vi "Dashboard Main.vi"() -> ()   [LabVIEW 2013]
uses:
  <vilib>/event_ctls.llb/eventvkey.ctl
  <vilib>/Rock Robotics/WPI/Dashboard/WPI_DashboardLogging Global.vi
  <vilib>/Utility/config.llb/Write Key (String).vi
  <vilib>/Utility/config.llb/Write Key (I32).vi
  <vilib>/Utility/config.llb/NI_LVConfig.lvlib
panel:
  out "Image Message":string="Timeout in Camera Communications"
  in  "Rec Mode":enum32{"Stop", "Record", "Playback"}(radio)
  in  "Dashboard Tab":T1(tab)
  in  "Camera Settings":T2={"Frame Rate"=30, "Compression"=30, "Size"=1} {"Frame Rate" scale=1.0..30.0; "Size" items=["640x480", "320x240", "160x120"]}
  out "MotorSliders R":cluster{"MotorSlide1":dbl, "MotorSlide2":dbl} {"MotorSlide2" scale=-1.0..1.0 scale format="%#_2e"; "MotorSlide1" scale=-1.0..1.0 scale format="%#_2e"}
  out "MotorChart R":cluster{"Numeric":dbl, "Numeric":dbl}(graph)
  out "MotorSliders L":T3 {"MotorSlide4 2" scale=0.0..14.0 scale format="%#_2e"; "MotorSlide2" scale=-1.0..1.0 scale format="%#_2e"; "MotorSlide1" scale=-1.0..1.0 scale format="%#_2e"}
  out "MotorChart L":T4(graph)
  out "JS1 Z":dbl(slide) scale=-1.0..1.0 scale format="%#_2e"
  out "Joystick 1":cluster{"X":dbl, "Y":dbl}[](graph)
  out "JS Buttons 1":T5
  out "JS2 Z":dbl(slide) scale=-1.0..1.0 scale format="%#_2e"
  out "Joystick 2":cluster{"X":dbl, "Y":dbl}[](graph)
  out "JS Buttons 2":T5
  out "Mode":T6(ring)=enum."Auto Disabled"
  out "Camera IP":string
  in  "DB Camera Config":bool
  out "fps":dbl format="%#.1g"
  out "Mbps":dbl format="%#.1g"
  out "Mbps 2":bool
  out "LED 1":bool
  in  "Slider 1":dbl(slide) scale=0.0..100.0
  in  "Checkbox 2":bool
  in  "Checkbox 1":bool
  in  "Test Slider":dbl(slide) scale=0.0..100.0 scale format="%#_3g"
  in  "On/Off":bool caption="Solenoid"
  in  "Test Name":u16(ring) items=["Select the test to run...", "Example Test", "-------------------------------", "List of tests is built in robot code.", "Replace with your own automated tests."]
  in  "Test Tree":string(tree)
  in  "Motor":cluster{"Value":dbl, "Enable":bool} {"Value" scale=-1.0..1.0 scale format="%#_3g"}
  out "Progress":T7 {"Test Progress" scale=0.0..100.0}
  in  "Rev/Fwd":cluster{"Forward":bool, "Reverse":bool}
  in  "Test Ring":u16(ring) items=["Auto", "Fixed indoor", "Fixed outdoor 1", "Fixed outdoor 2", "Fixed fluorescent 1", "Fixed fluorescent 2", "Hold current"]
  in  "Listbox":i32(listbox)
  out "Tree":string(tree)
  out "Camera Image":T8(plugin-control)
  in  "Enable":bool
  # "Left"
  # "Front"
  # "Right"
  # "Battery"
  # "Customize by placing controls and indicators here and name to\nmatch Dashboard Variables on robot."
  # "This tab is a great place for autonomous settings and validation.\nCustomize by placing controls and indicators here and name to\nmatch Dashboard Variables on robot."
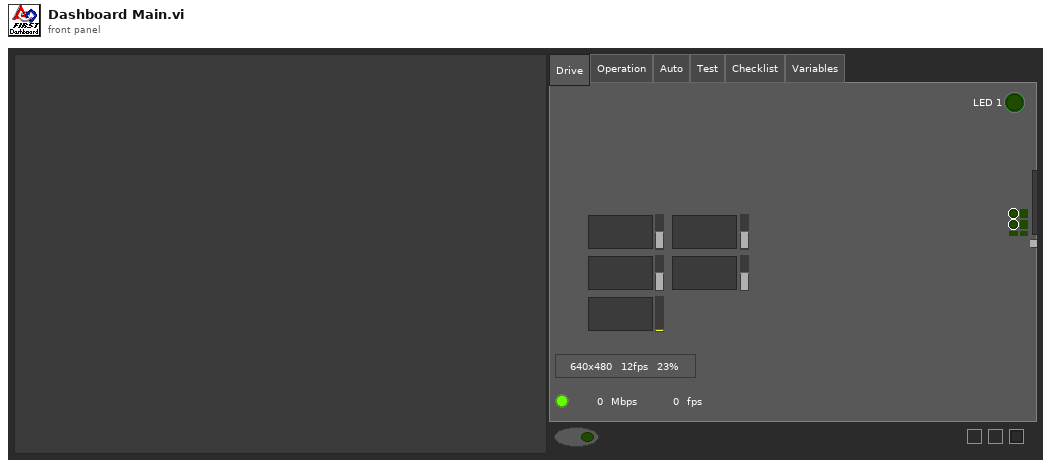
[diagram p1: front panel]
types:
  T1 = enum32{"Drive", "Operation", "Auto", "Test", "Checklist", "Variables"}
  T2 = cluster{"Frame Rate":i32, "Compression":i32, "Size":u16}
  T3 = cluster{"MotorSlide1":dbl, "MotorSlide2":dbl, "MotorSlide4 2":dbl}
  T4 = cluster{"Numeric":dbl, "Numeric":dbl, "Battery":sgl}
  T5 = cluster{bool, bool, bool, bool, bool, bool, bool, bool, bool, bool, bool, bool}
  T6 = enum8{"Tele-Op Disabled", "Tele-Op Enabled", "Auto Disabled", "Auto Enabled", "Test Disabled", "Test Enabled", ""}
  T7 = cluster{"Test Progress":u8, "Test Progress Text":string}
  T8 = typedef "IMAQ Image.ctl" = refnum<image>
  T9 = typedef "Image Type" = u32
  T10 = cluster{"Digital Inputs":bool[], "Digital Outputs":bool[]}
  T11 = cluster{"Competition mode":bool, "Robot Link":bool, "Autonomous":bool, "Enabled":bool, "E-Stop":bool, "Simulated":bool, "TestMode":bool, "Docked Window":bool}
  T12 = enum16{"0", "1", "2", "3", "4", "5", "6", "7", "8", "9", "A", "B", "C", "D", "E", "F", "G", "H", "I", "J", "K", "L", "M", "N", "O", "P", "Q", "R", "S", "T", "U", "V", "W", "X", "Y", "Z", "F1", "F2", "F3", "F4", "F5", "F6", "F7", "F8", "F9", "F10", "F11", "F12", "F13", "F14", "F15", "ADD", "BACK", "BACKSLASH", "CAPITAL", "COMMA", "DECIMAL", "DELETE", "DIVIDE", "DOWN", "END", "EQUALS", "ESCAPE", "GRAVE (`)", "HOME", "INSERT", "LBRACKET", "LCONTROL", "LEFT", "L ALT", "LSHIFT", "LWIN", "MINUS", "MULTIPLY", "NEXT", "NUMLOCK", "NUMPAD_0", "NUMPAD_1", "NUMPAD_2", "NUMPAD_3", "NUMPAD_4", "NUMPAD_5", "NUMPAD_6", "NUMPAD_7", "NUMPAD_8", "NUMPAD_9", "PAUSE", "PERIOD", "PRIOR (PG UP)", "RBRACKET", "RCONTROL", "RETURN", "RIGHT", "R ALT", "RSHIFT", "RWIN", "SCROLL", "SEMICOLON", "SLASH", "SPACE", "SUBTRACT", "TAB", "UP", "ENTER (num pad)", "' (quote)"}
  T13 = cluster{"Boolean Array[0]":bool, "Boolean Array[1]":bool, "Boolean Array[2]":bool, "Boolean Array[3]":bool, "Boolean Array[4]":bool, "Boolean Array[5]":bool, "Boolean Array[6]":bool, "Boolean Array[7]":bool, "Boolean Array[8]":bool, "Boolean Array[9]":bool, "Boolean Array[10]":bool, "Boolean Array[11]":bool}
  T14 = typedef "NI_LVConfig.lvlib/Config Data RefNum.ctl" = refnum<k1>
  T15 = typedef "eventvkey.ctl" = enum16{"ASCII", "Enter", "Return", "Shift", "Ctrl", "Alt", "Cmd", "Opt", "Caps", "NumLock", "Clear", "Break", "Up", "Down", "Left", "Right", "Insert", "Delete", "Home", "End", "PageUp", "PageDown", "Escape", "Help", "Pause", "ScrollLock", "F1", "F2", "F3", "F4", "F5", "F6", "F7", "F8", "F9", "F10", "F11", "F12", "F13", "F14", "F15", "F16", "F17", "F18", "F19", "F20", "F21", "F22", "F23", "F24", "Play", "VolumeUp", "VolumeDown", "Mute", "Two Byte Char"}
  T16 = cluster{"Image Size":bool, "Image Type":bool, "Pixel Value":bool, "ROI Information":bool, "Zoom Factor":bool}
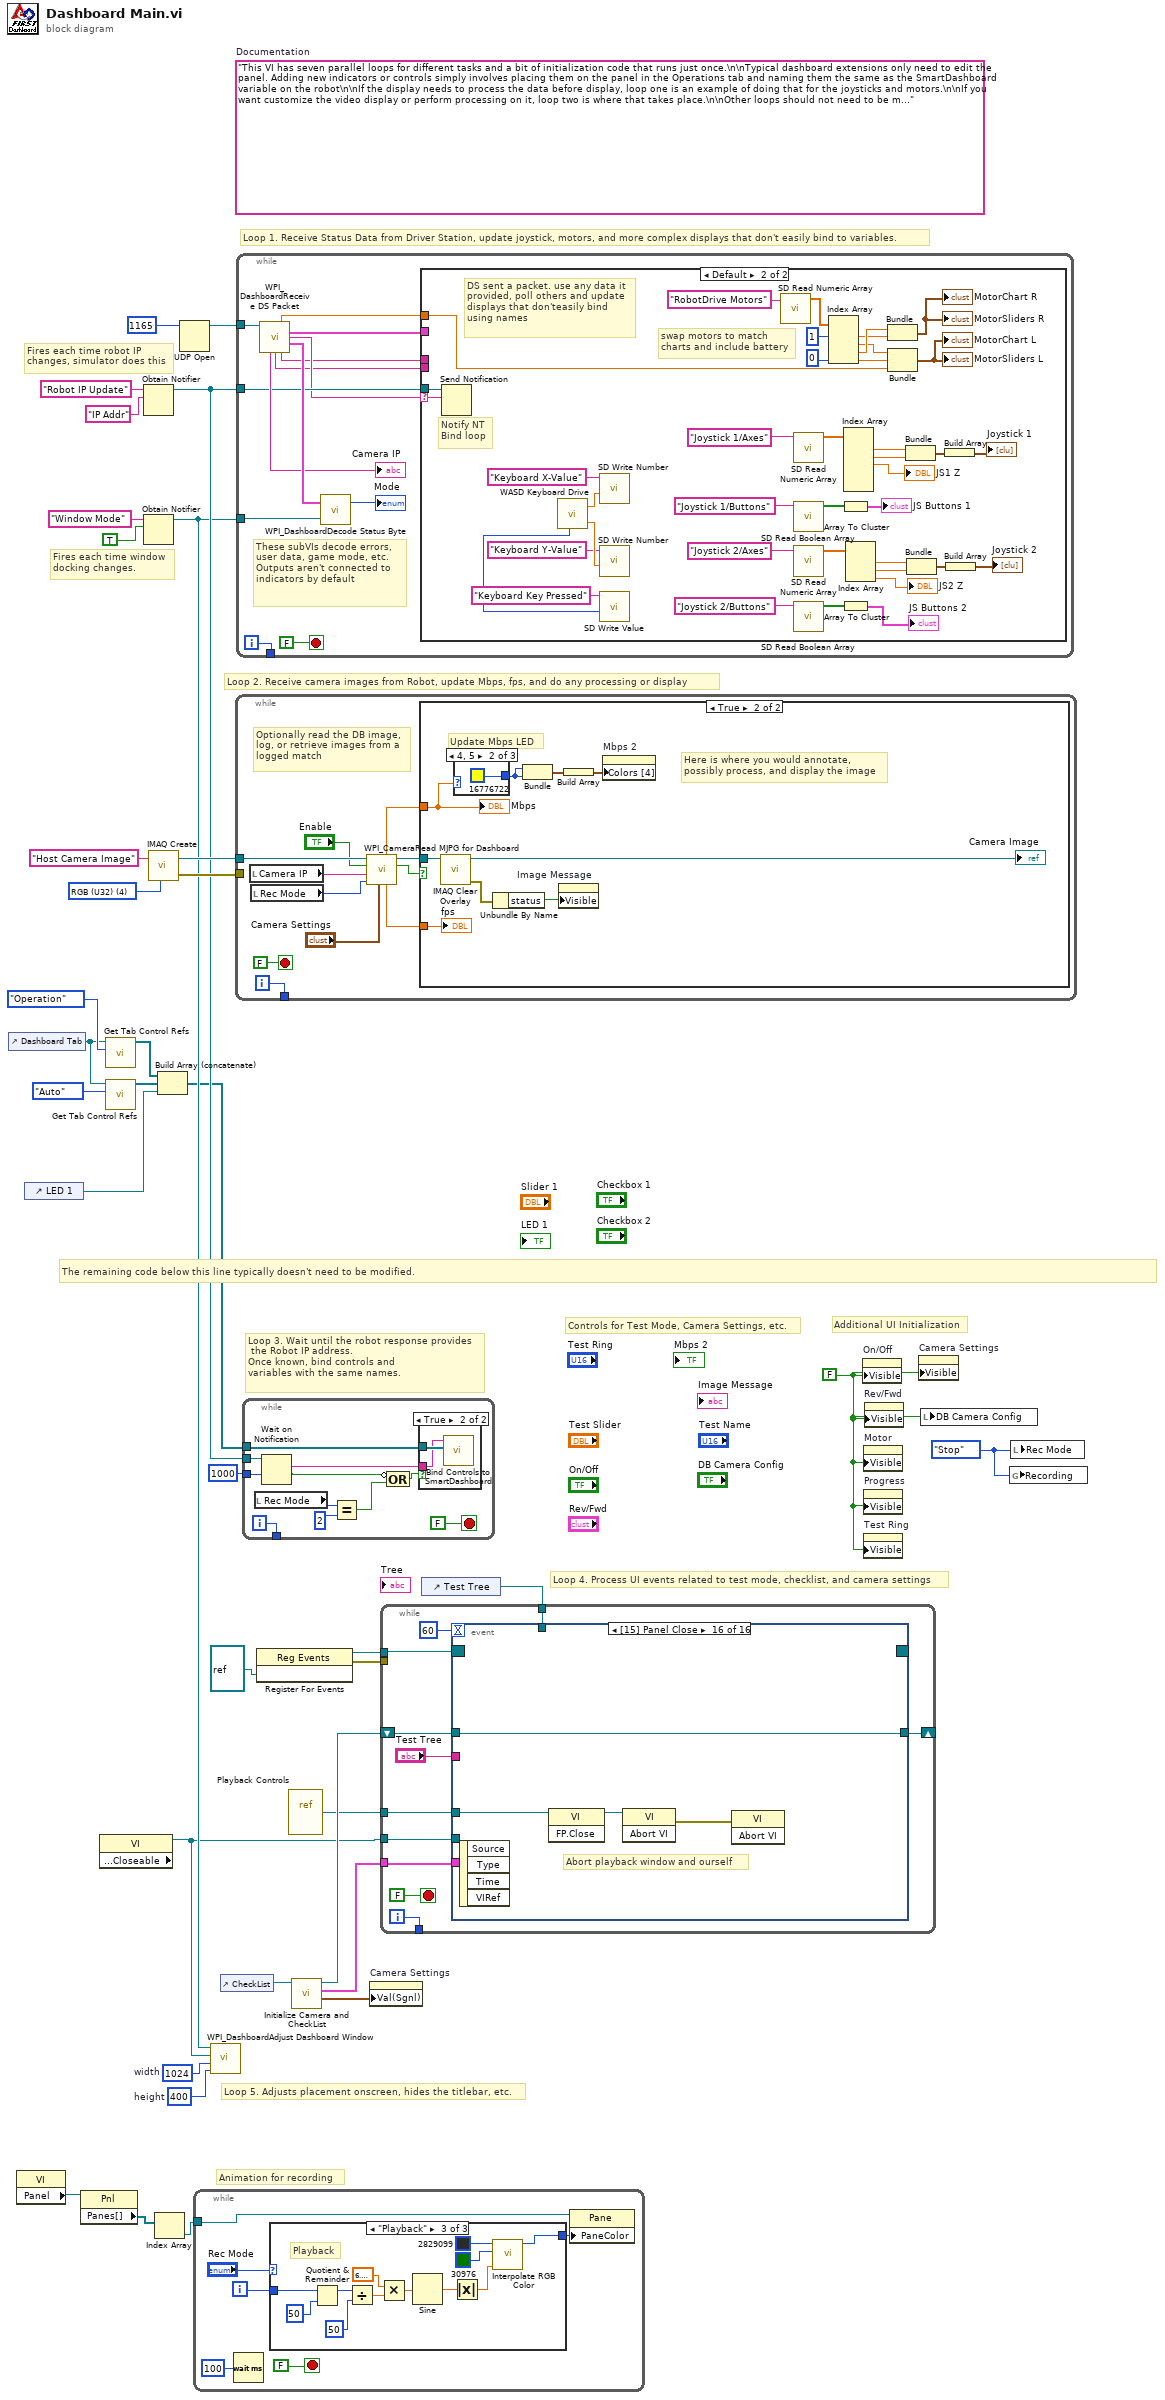
[diagram p0: block diagram]
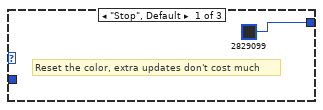
[diagram p2: hidden frame]
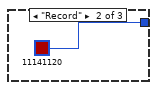
[diagram p3: hidden frame]
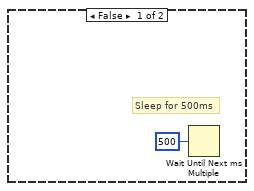
[diagram p5: hidden frame]
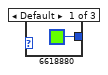
[diagram p6: hidden frame]
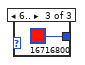
[diagram p7: hidden frame]
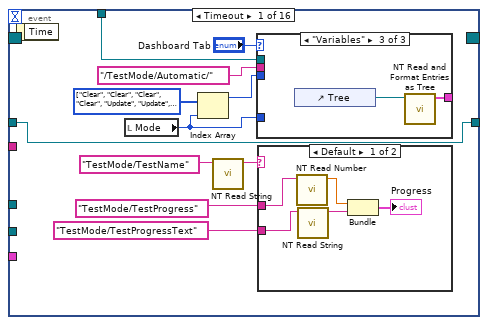
[diagram p8: hidden frame]
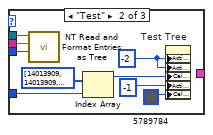
[diagram p10: hidden frame]
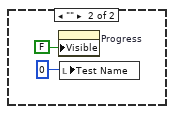
[diagram p11: hidden frame]
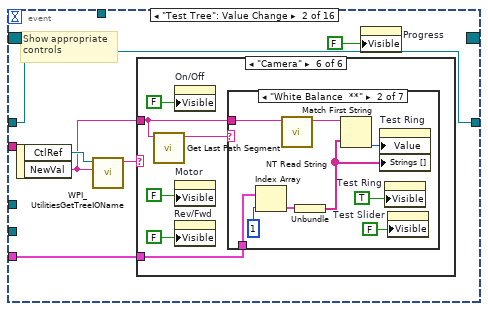
[diagram p12: hidden frame]
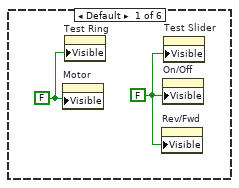
[diagram p13: hidden frame]
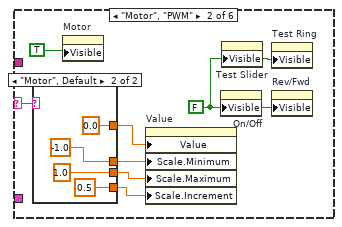
[diagram p14: hidden frame]
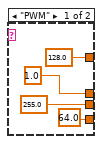
[diagram p15: hidden frame]
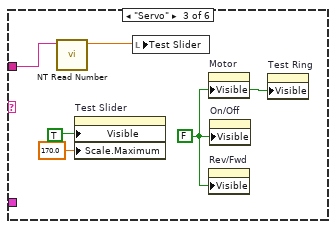
[diagram p16: hidden frame]
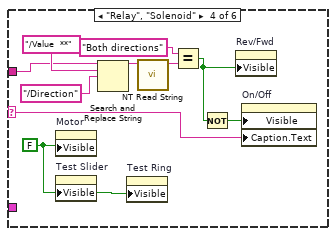
[diagram p17: hidden frame]
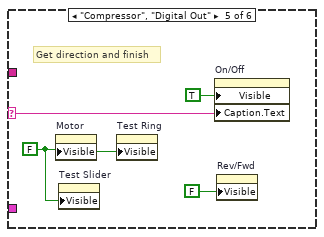
[diagram p18: hidden frame]
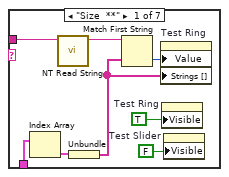
[diagram p19: hidden frame]
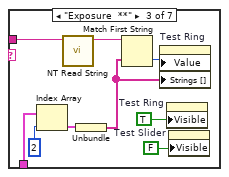
[diagram p20: hidden frame]
diagram:
  w8 = enum32{"Stop", "Record", "Playback"}."Stop" ("Rec Mode")
  w11 = 400  # height
  w12 = 1024  # width
  w25 = FALSE ("Visible")
  (unwired) "This VI has seven parallel loops for different tasks and a bit of initialization code that runs just once.\n\nTypical dashboard extensions only need to edit the panel. Adding new indicators or controls simply involves placing them on the panel in the Operations tab and naming them the same as the SmartDashboard variable on the robot\n\nIf the display needs to process the data before display, loop one is an example of doing that for the joysticks and motors.\n\nIf you want customize the video display or perform processing on it, loop two is where that takes place.\n\nOther loops should not need to be modified. They are pretty standard, and document the task they perform."  # Documentation
  w35 = T9 4 items=["Grayscale (U8)", "Grayscale (I16)", "Grayscale (SGL)", "Complex (CSG)", "RGB (U32)", "HSL (U32)", "RGB (U64)"] ("Image Type")
  # "Controls for Test Mode, Camera Settings, etc."
  # "Additional UI Initialization"
  # "Animation for recording"
  # "Fires each time robot IP\nchanges, simulator does this"
  # "Fires each time window\ndocking changes."
  # "The remaining code below this line typically doesn't need to be modified."
  # "Loop 4. Process UI events related to test mode, checklist, and camera settings"
  # "Loop 3. Wait until the robot response provides\n the Robot IP address.\nOnce known, bind controls and\nvariables with the same names."
  # "Loop 5. Adjusts placement onscreen, hides the titlebar, etc."
  # "Loop 1. Receive Status Data from Driver Station, update joystick, motors, and more complex displays that don't easily bind to variables."
  # "Loop 2. Receive camera images from Robot, update Mbps, fps, and do any processing or display"
  n1 = control-ref of="Dashboard Tab"() -> (w6:refnum<vi>)
  n2 = property class="VI"() -> ("Panel"=w19:refnum<vi>)  [unwired: 2 in, 2 out]
  n3 = control-ref of="LED 1"() -> (w1:refnum<vi>)
  n4 = property class="Pnl"(reference=w19) -> ("Panes[]"=w20:refnum<vi>[])  [unwired: 1 in, 2 out]
  n5 = property class="VI" props=["Front Panel.Closeable"]() -> (reference out=w7:refnum<vi>)  [unwired: 2 in, 2 out]
  n6 = call <vilib>:"Get Tab Control Refs.vi"("Page Index"=T1."Operation" ("Dashboard Tab"), "TabControl in"=w6) -> ("ControlsOnPage"=w4:refnum<vi>[])  [unwired: 9 in]
  n7 = call <vilib>:"Get Tab Control Refs.vi"("Page Index"=T1."Auto" ("Dashboard Tab"), "TabControl in"=w6) -> ("ControlsOnPage"=w5:refnum<vi>[])  [unwired: 9 in]
  n8 = Obtain Notifier(name (unnamed)="Robot IP Update", notification data type="IP Addr" ("name (unnamed)")) -> (notifier out=w29:refnum<notifier>)  [unwired: 2 in, 2 out]
  n9 = Obtain Notifier(name (unnamed)="Window Mode", notification data type=TRUE) -> (notifier out=w10:refnum<notifier>)  [unwired: 2 in, 2 out]
  n10 = call "IMAQ Create"("Image Name"="Host Camera Image", "Image Type"=w35) -> ("New Image"=w33:T8, "error out"=w32:errorcluster)  [unwired: 2 in, 1 out]
  n11 = Index Array(array=w20) -> (element=w18:refnum<vi>)  [unwired: 1 in]
  n12 = Build Array (concatenate)(w4, w5, w1) -> (w3:refnum<vi>[])
  n13 = UDP Open(11:u16 1165 ("port")) -> (port=w36:refnum<k16>)  [unwired: 2 in, 4 out]
  n14 = while {
    tunnel: w18 -> [w39]
    i -> [w42]
    stop <- FALSE stop-if-true
    n15 = Wait (ms)(milliseconds to wait=u32 100) -> ()  [unwired: 1 out]
    n16 = case shown="\"Playback\"" "Rec Mode" {
      tunnel: w42 -> [_ _ w57]
      tunnel: [u32 2829099 ("Base Color") u32 11141120 ("Target Color") w46] -> w38
      frame "Stop", Default {
        # "Reset the color, extra updates don't cost much"
      }
      frame "Record" {
      }
      frame "Playback" {
        # "Playback"
        n17 = Quotient & Remainder(x=w57, y=u32 50 ("milliseconds to wait")) -> (x-y*floor(x/y)=w53:u32)  [unwired: 1 out]
        n18 = Divide(x=w53, y=u32 50 ("milliseconds to wait")) -> (x/y=w50:dbl)
        n19 = Multiply(x=6.283185307179586, y=w50) -> (x*y=w55:dbl)
        n20 = Sine(x=w55) -> (sin(x)=w54:dbl)
        n21 = Absolute Value(x=w54) -> (abs(x)=w47:dbl)
        n22 = call "Interpolate RGB Color.vi"("Proportion"=w47, "Target Color"=u32 30976, "Base Color"=u32 2829099) -> ("Result Color"=w46:u32)  [unwired: 8 in]
      }
    }
    n23 = property class="Pane"(reference=w39, "PaneColor"=w38) -> ()  [unwired: 1 in, 2 out]
  }
  n24 = call <vilib>:"WPI_DashboardAdjust Dashboard Window.vi"("height"=w11, "width"=w12, "reference in"=w7, "Notifier in"=w10) -> ()  [unwired: 8 in]
  n25 = control-ref of="CheckList"() -> (w9:refnum<vi>)
  n26 = while {
    tunnel: w33 -> [w66]
    tunnel: w32 -> [_]
    tunnel: [w67] -> _
    i -> [w67]
    stop <- FALSE stop-if-true
    # "Optionally read the DB image,\nlog, or retrieve images from a\nlogged match"
    n27 = local read "Camera IP"() -> (w59:string)
    n28 = local read "Rec Mode"() -> (w58:enum32{"Stop", "Record", "Playback"})
    n29 = call <vilib>:"WPI_CameraRead MJPG for Dashboard.vi"("Camera Settings"="Camera Settings", "Rec Mode"=w58, "Camera IP"=w59, "Enable"="Enable", "Refnum in"=w66) -> ("Active"=w63:bool, "Refnum out"=w65:T8, "FPS"=w62:dbl, "Bandwidth (Mbps)"=w61:dbl)  [unwired: 3 in]
    n30 = case shown="True" w63 {
      tunnel: w65 -> [_ w73]
      tunnel: w61 -> [_ w72]
      tunnel: w62 -> [_ w70]
      frame False {
        # "Sleep for 500ms"
        n31 = Wait Until Next ms Multiple(millisecond multiple=u32 500) -> ()  [unwired: 1 out]
      }
      frame True {
        # "Here is where you would annotate,\npossibly process, and display the image"
        # "Update Mbps LED"
        n32 = call "IMAQ Clear Overlay"("Image"=w73) -> ("error out"=w77:errorcluster, "Image Out"=→"Camera Image":T8)  [unwired: 2 in, 7 out]
        n33 = case shown="4, 5" w72 {
          tunnel: [u32 6618880 ("Color Box") u32 16776722 ("Color Box") u32 16716800 ("Color Box")] -> w74
          frame Default {
          }
          frame 4, 5 {
          }
          frame 6.. {
          }
        }
        n34 = Unbundle By Name(w77) -> ("status"=w78:bool)
        n35 = Bundle("Color Box"=w74, "Color Box"=w74) -> (w76:cluster{"Color Box":u32, "Color Box":u32})  [unwired: 1 out]
        n36 = property on="Image Message" class="Str"("Visible"=w78) -> ()  [unwired: 2 in, 2 out]
        n37 = Build Array(w76) -> (w75:cluster{"Color Box":u32, "Color Box":u32}[])
        n38 = property on="Mbps 2" class="Bool (strict)"("Colors [4]"=w75) -> ()  [unwired: 2 in, 2 out]
        "Mbps" <- w72
        "fps" <- w70
      }
    }
  }
  n39 = while {
    tunnel: w36 -> [w92]
    tunnel: w29 -> [w87]
    tunnel: w10 -> [w91]
    tunnel: [w88] -> _
    i -> [w88]
    stop <- FALSE stop-if-true
    # "These subVIs decode errors, user data, game mode, etc.\nOutputs aren't connected to indicators by default"
    n40 = call <vilib>:"WPI_DashboardReceive DS Packet.vi"("Recv Socket"=w92) -> ("Battery"=w82:sgl, "Driver Station"=w83:T10, "Robot IP Address"=w86:string, "Status"=w93:T11, "Camera IP Address"=→"Camera IP":string, "Low Priority User Data"=w85:string, "High Priority User Data"=w84:string)  [unwired: 1 in, 7 out]
    n41 = call <vilib>:"WPI_DashboardDecode Status Byte.vi"("Window Mode Notifier"=w91, "Status"=w93) -> ("Mode"=→"Mode":T6)  [unwired: 1 out]
    n42 = case shown="Default" w86 {
      selector: w86 -> [_ w111]
      tunnel: w87 -> [_ w112]
      tunnel: w85 -> [_ _]
      tunnel: w84 -> [_ _]
      tunnel: w83 -> [_ _]
      tunnel: w82 -> [_ w110]
      frame "0.0.0.0" {
        # "DS not sending packets, or no robot exists yet.\nDon't poll the variables"
      }
      frame Default {
        # "Notify NT\nBind loop"
        # "DS sent a packet. use any data it\nprovided, poll others and update\ndisplays that don'teasily bind\nusing names"
        # "swap motors to match\ncharts and include battery"
        n43 = Send Notification(notification=w111, notifier=w112) -> ()  [unwired: 1 in, 2 out]
        n44 = call "WASD Keyboard Drive.vi"() -> ("Y-Axis"=w98:dbl, "X-Axis"=w100:dbl, "key"=w96:T12)  [unwired: 5 in]
        n45 = call <vilib>:"SD Write Number.vi"("Numeric"=w100, "Name"="Keyboard X-Value") -> ()  [unwired: 8 in, 2 out]
        n46 = call <vilib>:"SD Write Number.vi"("Numeric"=w98, "Name"="Keyboard Y-Value") -> ()  [unwired: 8 in, 2 out]
        n47 = call-poly <vilib>:"SD Write Value.vi"("Numeric"=w96, "Name"="Keyboard Key Pressed") -> ()  [unwired: 8 in, 2 out]
        n48 = call <vilib>:"SD Read Numeric Array.vi"("Name"="RobotDrive Motors") -> ("Numeric Array"=w109:dbl[])  [unwired: 8 in, 2 out]
        n49 = call <vilib>:"SD Read Numeric Array.vi"("Name"="Joystick 1/Axes") -> ("Numeric Array"=w128:dbl[])  [unwired: 8 in, 2 out]
        n50 = call <vilib>:"SD Read Boolean Array.vi"("Name"="Joystick 1/Buttons") -> ("Boolean Array"=w130:bool[])  [unwired: 8 in, 2 out]
        n51 = call <vilib>:"SD Read Numeric Array.vi"("Name"="Joystick 2/Axes") -> ("Numeric Array"=w122:dbl[])  [unwired: 8 in, 2 out]
        n52 = call <vilib>:"SD Read Boolean Array.vi"("Name"="Joystick 2/Buttons") -> ("Boolean Array"=w121:bool[])  [unwired: 8 in, 2 out]
        n53 = Index Array(array=w109, index #1=1, index #4=0) -> (element #1=w105:dbl, element #2=w104:dbl, element #3=w106:dbl, element #4=w101:dbl)  [unwired: 2 in]
        n54 = Array To Cluster(array=w130) -> (cluster=→"JS Buttons 1":T13)
        n55 = Array To Cluster(array=w121) -> (cluster=→"JS Buttons 2":T13)
        n56 = Index Array(array=w128) -> (element #1=w125:dbl, element #2=w126:dbl, element #3=→"JS1 Z":dbl)  [unwired: 6 in, 3 out]
        n57 = Index Array(array=w122) -> (element #1=w117:dbl, element #2=w116:dbl, element #3=→"JS2 Z":dbl)  [unwired: 3 in]
        n58 = Bundle("Numeric"=w106, "Numeric"=w105) -> (→"MotorChart R" →"MotorSliders R":cluster{"Numeric":dbl, "Numeric":dbl})  [unwired: 1 in]
        n59 = Bundle("Numeric"=w104, "Numeric"=w101, "Battery"=w110) -> (→"MotorChart L" →"MotorSliders L":T4)  [unwired: 1 in]
        n60 = Bundle("Numeric"=w125, "Numeric"=w126) -> (w124:cluster{"Numeric":dbl, "Numeric":dbl})  [unwired: 1 in]
        n61 = Bundle("Numeric"=w117, "Numeric"=w116) -> (w118:cluster{"Numeric":dbl, "Numeric":dbl})  [unwired: 1 in]
        n62 = Build Array(w124) -> (→"Joystick 1":cluster{"Numeric":dbl, "Numeric":dbl}[])
        n63 = Build Array(w118) -> (→"Joystick 2":cluster{"Numeric":dbl, "Numeric":dbl}[])
      }
    }
  }
  n64 = while {
    tunnel: w3 -> [w144]
    tunnel: w29 -> [w142]
    tunnel: [w140] -> _
    tunnel: u32 1000 ("milliseconds to wait") -> [w139]
    i -> [w140]
    stop <- FALSE stop-if-true
    n65 = local read "Rec Mode"() -> (w135:enum32{"Stop", "Record", "Playback"})
    n66 = Wait on Notification(notifier=w142, timeout in ms (-1)=w139) -> (notification=w141:string, timed out?=w137:bool)  [unwired: 2 in, 2 out]
    n67 = Equal?(x=w135, y=u16 2 ("Rec Mode")) -> (x = y?=w136:bool)
    n68 = Compound Arithmetic op=OR(invert w137, w136) -> (w138:bool)
    n69 = case shown="True" w138 {
      tunnel: w144 -> [_ w146]
      tunnel: w141 -> [_ w145]
      frame False {
      }
      frame True {
        n70 = call <vilib>:"Bind Controls to SmartDashboard.vi"("Bound Control Refs"=w146, "Server IP Address"=w145) -> ()  [unwired: 10 in]
      }
    }
  }
  n71 = register-events(refnum<vi> refnum) -> (reference out=w16:refnum<event-registration>, error out=w15:errorcluster)  [unwired: 2 in]
  n72 = vi-ref "Playback Controls.vi"() -> (w17:refnum<vi>)
  n73 = call "Initialize Camera and CheckList.vi"("ListBox in"=w9) -> ("Cluster"=w23:cluster{"value":i32, "value":i32, "index":i32}, "Array"=w24:cluster{string[]}[], "File Refnum"=w22:T14)  [unwired: 8 in]
  n74 = property on="Camera Settings" class="Clust (strict)"("Val(Sgnl)"=w23) -> ()  [unwired: 2 in, 2 out]
  n75 = control-ref of="Test Tree"() -> (w21:refnum<vi>)
  n76 = while {
    tunnel: w24 -> [w154]
    shift-right: [w153] -> _
    shift-left: w22 -> [w152]
    tunnel: [w151] -> _
    tunnel: w21 -> [w150]
    tunnel: w17 -> [w149]
    tunnel: w16 -> [w148]
    tunnel: w15 -> [_]
    tunnel: w7 -> [w147]
    i -> [w151]
    stop <- FALSE stop-if-true
    n77 = event shown="[15] Panel Close" {
      selector: w148 -> [_ _ _ _ _ _ _ _ _ _ _ _ _ _ _ _]
      dyn-events: [_ _ _ _ _ _ _ _ _ _ _ _ _ w392 _ _] -> _
      timeout: u32 60 ("milliseconds to wait") -> [_ _ _ _ _ _ _ _ _ _ _ _ _ _ _ _]
      tunnel: w150 -> [w164 _ _ _ _ _ _ _ _ _ _ _ _ _ _ _]
      tunnel: "Test Tree" -> [_ _ _ _ _ _ _ _ w361 w369 w371 w375 w383 _ _ _]
      tunnel: w154 -> [_ w188 _ _ _ _ w325 w355 _ _ _ _ _ _ _ _]
      tunnel: [w158 w187 w286 w291 w299 w311 w324 w348 w360 w367 w370 w374 w382 w394 w408 w409] -> w153
      tunnel: w152 -> [w158 w187 w286 w291 w299 w311 w323 w348 w360 w367 w370 w374 w382 w394 w408 w409]
      tunnel: w149 -> [_ _ _ _ _ _ _ _ _ _ _ _ _ w395 _ w412]
      tunnel: w147 -> [_ _ _ _ _ _ _ _ _ _ _ _ _ w390 _ _]
      event Timeout {
        w163 = enum16{"Update", "Clear"}[] [enum."Clear", enum."Clear", enum."Clear", enum."Clear", enum."Update", enum."Update", enum."Clear"] items=["Update", "Clear"]
        n78 = event-data() -> ()  [unwired: 1 in, 1 out]
        n79 = local read "Mode"() -> (w161:T6)
        n80 = Index Array(array=w163, index=w161) -> (element=w162:enum16{"Update", "Clear"})
        n81 = call <vilib>:"NT Read String.vi"("Name"="TestMode/TestName") -> ("String"=w167:string)  [unwired: 9 in, 1 out]
        n82 = case shown="\"Variables\"" "Dashboard Tab" {
          tunnel: w164 -> [_ w177 _]
          tunnel: "/TestMode/Automatic/" ("Name Pattern") -> [_ w176 _]
          tunnel: w162 -> [_ w175 _]
          tunnel: w161 -> [_ w173 _]
          tunnel: [_ _ w179] -> _
          frame "Operation", Default {
          }
          frame "Test" {
            w172 = -2 ("Active Item:Row Number")
            n83 = call <vilib>:"NT Read and Format Entries as Tree.vi"("Operation"=w175, "Name Pattern"=w176, "Tree Refnum"=w177) -> ()  [unwired: 7 in, 2 out]
            n84 = Index Array(array=u32[] [14013909, 14013909, 14013909, 14013909, 14013909, 16777215, 14013909], index=w173) -> (element=w171:u32)
            n85 = property on="Test Tree" class="Tree (strict)"("Active Item Row Number"=w172, "ActiveColNum"=w172, "CellBG"=w171, "Active Item Row Number"=-1 ("Active Item:Row Number"), "CellBG"=u32 5789784 ("Color Box")) -> ()  [unwired: 2 in, 2 out]
          }
          frame "Variables" {
            n86 = control-ref of="Tree"() -> (w178:refnum<vi>)
            n87 = call <vilib>:"NT Read and Format Entries as Tree.vi"("Tree Refnum"=w178) -> ("Formatted Strings"=w179:cluster{"Name":string, "Value":string}[])  [unwired: 9 in, 1 out]
          }
        }
        n88 = case shown="Default" w167 {
          tunnel: "TestMode/TestProgress" ("Name") -> [w181 _]
          tunnel: "TestMode/TestProgressText" ("Name") -> [w180 _]
          frame Default {
            n89 = call <vilib>:"NT Read Number.vi"("Name"=w181) -> ("Numeric"=w182:dbl)  [unwired: 9 in, 1 out]
            n90 = call <vilib>:"NT Read String.vi"("Name"=w180) -> ("String"=w183:string)  [unwired: 9 in, 1 out]
            n91 = Bundle("Numeric"=w182, "String"=w183) -> (→"Progress":cluster{"Numeric":dbl, "String":string})  [unwired: 1 in]
          }
          frame "" {
            n92 = property on="Progress" class="Clust (strict)"("Visible"=FALSE) -> ()  [unwired: 2 in, 2 out]
            n93 = local write "Test Name"(u16 0) -> ()
          }
        }
      }
      event "Test Tree": Value Change {
        # "Show appropriate\ncontrols"
        n94 = event-data() -> ("CtlRef"=w191:refnum<vi>, "NewVal"=w189:string)  [unwired: 1 in]
        n95 = call <vilib>:"WPI_UtilitiesGetTreeIOName.vi"("NewVal"=w189, "TreeControl in"=w191) -> ("I/O Name"=w192:string)  [unwired: 9 in]
        n96 = case shown="\"Camera\"" w192 {
          selector: w192 -> [_ w199 _ w217 w226 _]
          tunnel: w189 -> [_ _ w214 w216 _ w233]
          tunnel: w188 -> [_ _ _ _ _ w232]
          frame Default {
            w194 = FALSE ("Visible")
            w193 = FALSE ("Visible")
            n97 = property on="Motor" class="Clust (strict)"("Visible"=w193) -> ()  [unwired: 2 in, 2 out]
            n98 = property on="Test Ring" class="Ring (strict)"("Visible"=w193) -> ()  [unwired: 2 in, 2 out]
            n99 = property on="Rev/Fwd" class="Clust (strict)"("Visible"=w194) -> ()  [unwired: 2 in, 2 out]
            n100 = property on="On/Off" class="Bool (strict)"("Visible"=w194) -> ()  [unwired: 2 in, 2 out]
            n101 = property on="Test Slider" class="Slide (strict)"("Visible"=w194) -> ()  [unwired: 2 in, 2 out]
          }
          frame "Motor", "PWM" {
            w200 = FALSE ("Visible")
            n102 = case shown="\"Motor\", Default" w199 {
              tunnel: [1.0 ("Value") -1.0 ("Value")] -> w198
              tunnel: [255.0 ("Value") 1.0 ("Value")] -> w197
              tunnel: [128.0 ("Value") 0.0 ("Value")] -> w196
              tunnel: [64.0 ("Value") 0.5 ("Value")] -> w195
              frame "PWM" {
              }
              frame "Motor", Default {
              }
            }
            n103 = property on="Motor" class="Clust (strict)"("Visible"=TRUE) -> ()  [unwired: 2 in, 2 out]
            n104 = property on="Value" class="Slide (strict)"("Value"=w196, "Scale.Minimum"=w198, "Scale.Maximum"=w197, "Scale.Increment"=w195) -> ()  [unwired: 2 in, 2 out]
            n105 = property on="On/Off" class="Bool (strict)"("Visible"=w200) -> ()  [unwired: 2 in, 2 out]
            n106 = property on="Test Slider" class="Slide (strict)"("Visible"=w200) -> ()  [unwired: 2 in, 2 out]
            n107 = property on="Test Ring" class="Ring (strict)"("Visible"=w200) -> ()  [unwired: 2 in, 2 out]
            n108 = property on="Rev/Fwd" class="Clust (strict)"("Visible"=w200) -> ()  [unwired: 2 in, 2 out]
          }
          frame "Servo" {
            w212 = FALSE ("Visible")
            n109 = call <vilib>:"NT Read Number.vi"("Name"=w214) -> ("Numeric"=w213:dbl)  [unwired: 9 in, 1 out]
            n110 = property on="Test Slider" class="Slide (strict)"("Visible"=TRUE, "Scale.Maximum"=170.0 ("Scale.Range:Maximum")) -> ()  [unwired: 2 in, 2 out]
            n111 = local write "Test Slider"(w213) -> ()
            n112 = property on="Motor" class="Clust (strict)"("Visible"=w212) -> ()  [unwired: 2 in, 2 out]
            n113 = property on="Rev/Fwd" class="Clust (strict)"("Visible"=w212) -> ()  [unwired: 2 in, 2 out]
            n114 = property on="On/Off" class="Bool (strict)"("Visible"=w212) -> ()  [unwired: 2 in, 2 out]
            n115 = property on="Test Ring" class="Ring (strict)"("Visible"=w212) -> ()  [unwired: 2 in, 2 out]
          }
          frame "Relay", "Solenoid" {
            w215 = FALSE ("Visible")
            n116 = property on="Motor" class="Clust (strict)"("Visible"=w215) -> ()  [unwired: 2 in, 2 out]
            n117 = property on="Test Slider" class="Slide (strict)"("Visible"=w215) -> ()  [unwired: 2 in, 2 out]
            n118 = Search and Replace String(input string=w216, search string="/Value  **", replace string="/Direction") -> (result string=w222:string)  [unwired: 5 in, 3 out]
            n119 = property on="Test Ring" class="Ring (strict)"("Visible"=w215) -> ()  [unwired: 2 in, 2 out]
            n120 = call <vilib>:"NT Read String.vi"("Name"=w222) -> ("String"=w220:string)  [unwired: 9 in, 1 out]
            n121 = Equal?(x="Both directions", y=w220) -> (x = y?=w218:bool)
            n122 = Not(x=w218) -> (.not. x?=w219:bool)
            n123 = property on="Rev/Fwd" class="Clust (strict)"("Visible"=w218) -> ()  [unwired: 2 in, 2 out]
            n124 = property on="On/Off" class="Bool (strict)"("Visible"=w219, "Caption.Text"=w217) -> ()  [unwired: 2 in, 2 out]
          }
          frame "Compressor", "Digital Out" {
            w225 = FALSE ("Visible")
            # "Get direction and finish"
            n125 = property on="Motor" class="Clust (strict)"("Visible"=w225) -> ()  [unwired: 2 in, 2 out]
            n126 = property on="Test Slider" class="Slide (strict)"("Visible"=w225) -> ()  [unwired: 2 in, 2 out]
            n127 = property on="Test Ring" class="Ring (strict)"("Visible"=w225) -> ()  [unwired: 2 in, 2 out]
            n128 = property on="On/Off" class="Bool (strict)"("Visible"=TRUE, "Caption.Text"=w226) -> ()  [unwired: 2 in, 2 out]
            n129 = property on="Rev/Fwd" class="Clust (strict)"("Visible"=FALSE) -> ()  [unwired: 2 in, 2 out]
          }
          frame "Camera" {
            n130 = call <vilib>:"Get Last Path Segment.vi"("String in"=w233) -> ("String out"=w234:string)  [unwired: 10 in]
            n131 = property on="On/Off" class="Bool (strict)"("Visible"=FALSE) -> ()  [unwired: 2 in, 2 out]
            n132 = property on="Motor" class="Clust (strict)"("Visible"=FALSE) -> ()  [unwired: 2 in, 2 out]
            n133 = property on="Rev/Fwd" class="Clust (strict)"("Visible"=FALSE) -> ()  [unwired: 2 in, 2 out]
            n134 = case shown="\"White Balance  **\"" w234 {
              tunnel: w233 -> [w240 w249 w258 w267 w276 _ w282]
              tunnel: w232 -> [w238 w246 w255 w264 w273 _ _]
              frame "Size  **" {
                n135 = Index Array(array=w238) -> (element=w237:cluster{string[]})  [unwired: 1 in]
                n136 = call <vilib>:"NT Read String.vi"("Name"=w240) -> ("String"=w239:string)  [unwired: 9 in, 1 out]
                n137 = Unbundle(w237) -> (w235:string[])
                n138 = Match First String(2:w235, 3:w239) -> (0:w236:i32)  [unwired: 1 out]
                n139 = property on="Test Ring" class="Ring (strict)"("Value"=w236, "Strings []"=w235) -> ()  [unwired: 2 in, 2 out]
                n140 = property on="Test Ring" class="Ring (strict)"("Visible"=TRUE) -> ()  [unwired: 2 in, 2 out]
                n141 = property on="Test Slider" class="Slide (strict)"("Visible"=FALSE) -> ()  [unwired: 2 in, 2 out]
              }
              frame "White Balance  **" {
                n142 = Index Array(array=w246, index=1) -> (element=w247:cluster{string[]})
                n143 = call <vilib>:"NT Read String.vi"("Name"=w249) -> ("String"=w248:string)  [unwired: 9 in, 1 out]
                n144 = Unbundle(w247) -> (w244:string[])
                n145 = Match First String(2:w244, 3:w248) -> (0:w243:i32)  [unwired: 1 out]
                n146 = property on="Test Ring" class="Ring (strict)"("Value"=w243, "Strings []"=w244) -> ()  [unwired: 2 in, 2 out]
                n147 = property on="Test Ring" class="Ring (strict)"("Visible"=TRUE) -> ()  [unwired: 2 in, 2 out]
                n148 = property on="Test Slider" class="Slide (strict)"("Visible"=FALSE) -> ()  [unwired: 2 in, 2 out]
              }
              frame "Exposure  **" {
                n149 = Index Array(array=w255, index=2) -> (element=w256:cluster{string[]})
                n150 = call <vilib>:"NT Read String.vi"("Name"=w258) -> ("String"=w257:string)  [unwired: 9 in, 1 out]
                n151 = Unbundle(w256) -> (w252:string[])
                n152 = Match First String(2:w252, 3:w257) -> (0:w253:i32)  [unwired: 1 out]
                n153 = property on="Test Ring" class="Ring (strict)"("Value"=w253, "Strings []"=w252) -> ()  [unwired: 2 in, 2 out]
                n154 = property on="Test Ring" class="Ring (strict)"("Visible"=TRUE) -> ()  [unwired: 2 in, 2 out]
                n155 = property on="Test Slider" class="Slide (strict)"("Visible"=FALSE) -> ()  [unwired: 2 in, 2 out]
              }
              frame "Exposure Priority  **" {
                n156 = Index Array(array=w264, index=3) -> (element=w265:cluster{string[]})
                n157 = call <vilib>:"NT Read String.vi"("Name"=w267) -> ("String"=w266:string)  [unwired: 9 in, 1 out]
                n158 = Unbundle(w265) -> (w261:string[])
                n159 = Match First String(2:w261, 3:w266) -> (0:w262:i32)  [unwired: 1 out]
                n160 = property on="Test Ring" class="Ring (strict)"("Value"=w262, "Strings []"=w261) -> ()  [unwired: 2 in, 2 out]
                n161 = property on="Test Ring" class="Ring (strict)"("Visible"=TRUE) -> ()  [unwired: 2 in, 2 out]
                n162 = property on="Test Slider" class="Slide (strict)"("Visible"=FALSE) -> ()  [unwired: 2 in, 2 out]
              }
              frame "Color Enable  **" {
                n163 = Index Array(array=w273, index=4) -> (element=w274:cluster{string[]})
                n164 = call <vilib>:"NT Read String.vi"("Name"=w276) -> ("String"=w275:string)  [unwired: 9 in, 1 out]
                n165 = Unbundle(w274) -> (w270:string[])
                n166 = Match First String(2:w270, 3:w275) -> (0:w271:i32)  [unwired: 1 out]
                n167 = property on="Test Ring" class="Ring (strict)"("Value"=w271, "Strings []"=w270) -> ()  [unwired: 2 in, 2 out]
                n168 = property on="Test Ring" class="Ring (strict)"("Visible"=TRUE) -> ()  [unwired: 2 in, 2 out]
                n169 = property on="Test Slider" class="Slide (strict)"("Visible"=FALSE) -> ()  [unwired: 2 in, 2 out]
              }
              frame Default {
                n170 = property on="Test Ring" class="Ring (strict)"("Visible"=FALSE) -> ()  [unwired: 2 in, 2 out]
                n171 = property on="Test Slider" class="Slide (strict)"("Visible"=FALSE) -> ()  [unwired: 2 in, 2 out]
              }
              frame "Brightness  **", "Color Level  **", "Compression  **", "FPS  **", "Sharpness  **" {
                n172 = call <vilib>:"NT Read Number.vi"("Name"=w282) -> ("Numeric"=w281:dbl)  [unwired: 9 in, 1 out]
                n173 = local write "Test Slider"(w281) -> ()
                n174 = property on="Test Slider" class="Slide (strict)"("Visible"=TRUE, "Scale.Maximum"=100.0 ("Scale.Range:Maximum")) -> ()  [unwired: 2 in, 2 out]
                n175 = property on="Test Ring" class="Ring (strict)"("Visible"=FALSE) -> ()  [unwired: 2 in, 2 out]
              }
            }
          }
        }
        n176 = property on="Progress" class="Clust (strict)"("Visible"=FALSE) -> ()  [unwired: 2 in, 2 out]
      }
      event "Test Name": Mouse Enter {
        # "Populate the ring with the list of tests"
        n177 = event-data() -> ()  [unwired: 1 in, 1 out]
        n178 = call <vilib>:"NT Read String Array.vi"("Name"="TestMode/TestList") -> ("String Array"=w290:string[])  [unwired: 9 in, 1 out]
        n179 = Build Array (concatenate)("Select the test to run...", w290) -> (w289:string[])
        n180 = property on="Test Name" class="Ring (strict)"("Strings []"=w289) -> ()  [unwired: 2 in, 2 out]
      }
      event "Test Name": Value Change {
        w292 = FALSE ("Visible")
        # "Tell the robot the test name to run"
        n181 = event-data() -> ("NewVal"=w296:u16)  [unwired: 1 in]
        n182 = property on="Test Name" class="Ring (strict)"() -> ("Strings []"=w297:string[])  [unwired: 2 in, 2 out]
        n183 = local write "Progress"(T7 {"Test Progress"=0, "Test Progress Text"=""} ("Progress")) -> ()
        n184 = Index Array(array=w297, index=w296) -> (element=w295:string)
        n185 = call <vilib>:"NT Write String.vi"("String"=w295, "Name"="TestMode/TestName") -> ()  [unwired: 9 in, 1 out]
        n186 = property on="Progress" class="Clust (strict)"("Visible"=TRUE) -> ()  [unwired: 2 in, 2 out]
        n187 = property on="Motor" class="Clust (strict)"("Visible"=w292) -> ()  [unwired: 2 in, 2 out]
        n188 = property on="Test Slider" class="Slide (strict)"("Visible"=w292) -> ()  [unwired: 2 in, 2 out]
        n189 = property on="On/Off" class="Bool (strict)"("Visible"=w292) -> ()  [unwired: 2 in, 2 out]
        n190 = property on="Rev/Fwd" class="Clust (strict)"("Visible"=w292) -> ()  [unwired: 2 in, 2 out]
        n191 = property on="Test Ring" class="Ring (strict)"("Visible"=w292) -> ()  [unwired: 2 in, 2 out]
      }
      event "Listbox": Double Click {
        n192 = event-data() -> ("PlatMods.Shift"=w300:bool, "Row"=w302:i32)  [unwired: 1 in]
        n193 = case shown="True" w300 {
          tunnel: w302 -> [w306 _]
          tunnel: 1 -> [w305 _]
          frame False {
            n194 = property on="Listbox" class="LstBox (strict)"() -> ("Item Symbols"=w304:i32[])  [unwired: 2 in, 2 out]
            n195 = Replace Array Subset(array=w304, new element=w305, index=w306) -> (w303:i32[])
            n196 = property on="Listbox" class="LstBox (strict)"("Item Symbols"=w303) -> ()  [unwired: 2 in, 2 out]
          }
          frame True {
            w307 = 0 ("Top Row")
            n197 = property on="Listbox" class="LstBox (strict)"() -> ("Number of Rows"=w309:u32)  [unwired: 2 in, 2 out]
            n198 = Initialize Array(0, w309) -> (w308:i32[])
            n199 = property on="Listbox" class="LstBox (strict)"("Top Row"=w307, "Value"=w307, "Item Symbols"=w308) -> ()  [unwired: 2 in, 2 out]
          }
        }
      }
      event "Listbox": Key Down {
        n200 = event-data() -> ("VKey"=w313:T15)  [unwired: 1 in]
        n201 = case shown="\"Left\", \"Right\"" w313 {
          selector: w313 -> [w318 _]
          tunnel: eventvkey."Left" ("VKey") -> [w316 _]
          frame "Left", "Right" {
            n202 = Equal?(x=w316, y=w318) -> (x = y?=w317:bool)
            n203 = Select(t=0, s=w317, f=1) -> (s? t:f=w319:i32)
            n204 = property on="Listbox" class="LstBox (strict)"() -> ("Item Symbols"=w322:i32[])  [unwired: 2 in, 2 out]
            n205 = Replace Array Subset(array=w322, new element=w319, index="Listbox") -> (w321:i32[])
            n206 = property on="Listbox" class="LstBox (strict)"("Item Symbols"=w321) -> ()  [unwired: 2 in, 2 out]
          }
          frame Default {
          }
        }
      }
      event "DB Camera Config": Value Change {
        n207 = event-data() -> ("NewVal"=w326:bool)  [unwired: 1 in]
        n208 = case shown="False" w326 {
          tunnel: w325 -> [w335 _]
          tunnel: [w328 w346] -> w324
          tunnel: w323 -> [w327 w346]
          frame False {
            w342 = "Camera"
            w345 = FALSE ("Visible")
            n209 = local read "Camera Settings"() -> (w334:T2)
            n210 = Index Array(array=w335) -> (element=w338:cluster{string[]})  [unwired: 1 in]
            n211 = Unbundle(w334) -> ("Frame Rate"=w333:i32, "Compression"=w332:i32, "Size"=w336:u16)
            n212 = Unbundle(w338) -> (w337:string[])
            n213 = Index Array(array=w337, index=w336) -> (element=w331:string)
            n214 = call-poly <vilib>:"Write Key.vi"("section"=w342, "value"=w331, "key"="Size", "refnum"=w327) -> ("refnum out"=w344:T14)  [unwired: 2 in, 5 out]
            n215 = call-poly <vilib>:"Write Key.vi"("section"=w342, "value"=w333, "key"="FrameRate", "refnum"=w344) -> ("refnum out"=w343:T14)  [unwired: 1 in, 6 out]
            n216 = property on="Camera Settings" class="Clust (strict)"("Visible"=w345) -> ()  [unwired: 2 in, 2 out]
            n217 = local write "DB Camera Config"(w345) -> ()
            n218 = call-poly <vilib>:"Write Key.vi"("section"=w342, "value"=w332, "key"="Compression", "refnum"=w343) -> ("refnum out"=w329:T14)  [unwired: 1 in, 6 out]
            n219 = call <vilib>:"Close Config Data.vi"("refnum"=w329) -> ("file path"=w330:path)  [unwired: 2 in, 8 out]
            n220 = call <vilib>:"Open Config Data.vi"("configuration file path"=w330) -> ("refnum"=w328:T14)  [unwired: 8 in, 2 out]
          }
          frame True {
            n221 = property on="Camera Settings" class="Clust (strict)"("Visible"=TRUE) -> ()  [unwired: 2 in, 2 out]
          }
        }
      }
      event "Camera Settings": Value Change {
        n222 = event-data() -> ("NewVal"=w359:T2)  [unwired: 1 in]
        n223 = Index Array(array=w355) -> (element=w354:cluster{string[]})  [unwired: 1 in]
        n224 = Unbundle(w359) -> ("Frame Rate"=w350:i32, "Compression"=w349:i32, "Size"=w352:u16)
        n225 = Unbundle(w354) -> (w353:string[])
        n226 = Index Array(array=w353, index=w352) -> (element=w351:string)
        n227 = Format Into String(format string="%s   %dfps   %d%%", w351, w350, w349) -> (resulting string=w356:string)  [unwired: 2 in, 1 out]
        n228 = Build Array(w356) -> (w357:string[])
        n229 = property on="DB Camera Config" class="Bool (strict)"("Strings [4]"=w357) -> ()  [unwired: 2 in, 2 out]
      }
      event "Motor.Enable": Value Change {
        n230 = event-data() -> ("NewVal"=w365:bool)  [unwired: 1 in]
        n231 = Unbundle("Motor") -> ("Value"=w364:dbl)  [unwired: 1 out]
        n232 = Select(t=w364, s=w365, f=0.0) -> (s? t:f=w362:dbl)
        n233 = call <vilib>:"NT Write Number.vi"("Numeric"=w362, "Name"=w361) -> ()  [unwired: 9 in, 1 out]
      }
      event "Test Slider": Value Change {
        n234 = event-data() -> ("NewVal"=w368:dbl)  [unwired: 1 in]
        n235 = call <vilib>:"NT Write Number.vi"("Numeric"=w368, "Name"=w369) -> ()  [unwired: 9 in, 1 out]
      }
      event "On/Off": Value Change {
        n236 = event-data() -> ("NewVal"=w373:bool)  [unwired: 1 in]
        n237 = Boolean To (0,1)(Boolean=w373) -> (0, 1=w372:i16)
        n238 = call <vilib>:"NT Write Number.vi"("Numeric"=w372, "Name"=w371) -> ()  [unwired: 9 in, 1 out]
      }
      event "Rev/Fwd": Value Change {
        n239 = event-data() -> ("NewVal.Forward"=w381:bool, "NewVal.Reverse"=w380:bool)  [unwired: 1 in]
        n240 = Boolean To (0,1)(Boolean=w381) -> (0, 1=w377:i16)
        n241 = Boolean To (0,1)(Boolean=w380) -> (0, 1=w379:i16)
        n242 = Negate(x=w379) -> (-x=w378:i16)
        n243 = Add(x=w377, y=w378) -> (x+y=w376:i16)
        n244 = call <vilib>:"NT Write Number.vi"("Numeric"=w376, "Name"=w375) -> ()  [unwired: 9 in, 1 out]
      }
      event "Test Ring": Value Change {
        n245 = event-data() -> ("NewVal"=w385:u16)  [unwired: 1 in]
        n246 = property on="Test Ring" class="Ring (strict)"() -> ("Strings []"=w386:string[])  [unwired: 2 in, 2 out]
        n247 = Index Array(array=w386, index=w385) -> (element=w384:string)
        n248 = call <vilib>:"NT Write String.vi"("String"=w384, "Name"=w383) -> ()  [unwired: 9 in, 1 out]
      }
      event "Rec Mode": Value Change {
        # "Update globals for recording mode and path to read log from.\nClear when logging and let NetworkTables set path for vision to\nuse."
        n249 = event-data() -> ("NewVal"=w396:enum32{"Stop", "Record", "Playback"})  [unwired: 1 in]
        n250 = global write "WPI_DashboardLogging Global.vi" "Logging Filename"(path "") -> ()
        n251 = case shown="\"Stop\", \"Record\"" w396 {
          tunnel: w395 -> [_ w398 w406]
          tunnel: [_ _ w405] -> w392
          tunnel: [_ _ w404] -> _
          tunnel: w390 -> [_ _ w402]
          tunnel: cluster{i32, i32} {-250, 170} -> [_ _ w401]
          tunnel: [_ _ T16 {"Image Size"=TRUE, "Image Type"=TRUE, "Pixel Value"=TRUE, "ROI Information"=TRUE, "Zoom Factor"=FALSE} ("Image Information Shown:All Elements")] -> w388
          tunnel: [_ _ TRUE ("Zoom Factor")] -> w387
          frame Default {
          }
          frame "Stop", "Record" {
            # "Place Window too"
            n252 = invoke class="VI" method="FP.Close"(reference=w398) -> (reference out=w397:refnum<vi>)  [unwired: 2 in, 2 out]
            n253 = invoke class="VI" method="Abort VI"(reference=w397) -> ()  [unwired: 2 in, 3 out]
          }
          frame "Playback" {
            n254 = call "Open Playback Panel.vi"("Offset"=w401, "DB VI Ref"=w402, "Playback in"=w406) -> ("Playback out"=w403:refnum<vi>)  [unwired: 8 in]
            n255 = register-events(w403) -> (reference out=w405:refnum<event-registration>, error out=w404:errorcluster)  [unwired: 2 in]
          }
        }
        n256 = global write "WPI_DashboardLogging Global.vi" "Recording"(w396) -> ()
        n257 = property on="Camera Image" class="ImageControl"("Image Information Shown"=w388, "Image Information Visible"=w387) -> ()  [unwired: 2 in, 2 out]
        n258 = call <vilib>:"WPI_DashboardNT Log FieldName Cache.vi"("Operation"=enum16{"Lookup/Add", "Index", "Clear"}."Clear") -> ()  [unwired: 8 in, 3 out]
      }
      event Panel Close {
        w407 = enum32{"Stop", "Record", "Playback"}."Stop" ("Rec Mode")
        n259 = event-data() -> ()  [unwired: 1 in, 4 out]
        n260 = local write "Rec Mode"(w407) -> ()
        n261 = global write "WPI_DashboardLogging Global.vi" "Recording"(w407) -> ()
      }
      event Panel Close {
        # "Abort playback window and ourself"
        n262 = event-data() -> ()  [unwired: 1 in, 4 out]
        n263 = invoke class="VI" method="FP.Close"(reference=w412) -> (reference out=w411:refnum<vi>)  [unwired: 2 in, 2 out]
        n264 = invoke class="VI" method="Abort VI"(reference=w411) -> (error out=w410:errorcluster)  [unwired: 2 in, 2 out]
        n265 = invoke class="VI" method="Abort VI"(error in=w410) -> ()  [unwired: 2 in, 3 out]
      }
    }
  }
  n266 = property on="On/Off" class="Bool (strict)"("Visible"=w25) -> ()  [unwired: 2 in, 2 out]
  n267 = property on="Motor" class="Clust (strict)"("Visible"=w25) -> ()  [unwired: 2 in, 2 out]
  n268 = property on="Progress" class="Clust (strict)"("Visible"=w25) -> ()  [unwired: 2 in, 2 out]
  n269 = property on="Test Ring" class="Ring (strict)"("Visible"=w25) -> ()  [unwired: 2 in, 2 out]
  n270 = property on="Rev/Fwd" class="Clust (strict)"("Visible"=w25) -> ()  [unwired: 2 in, 2 out]
  n271 = property on="Camera Settings" class="Clust (strict)"("Visible"=w25) -> ()  [unwired: 2 in, 2 out]
  n272 = local write "DB Camera Config"(w25) -> ()
  n273 = global write "WPI_DashboardLogging Global.vi" "Recording"(w8) -> ()
  n274 = local write "Rec Mode"(w8) -> ()
